vi "DeviceNet.vi"(0 "CloseVi?":bool) -> ()   [LabVIEW 2011]
uses:
  GlobalVariables.vi
panel:
  in  "DNET3_3":u8
  in  "DNET3_2":u8
  in  "DNET3_1":u8
  in  "DNET3_0":u8
  in  "DNET2_3":u8
  in  "DNET2_2":u8
  in  "DNET2_1":u8
  in  "DNET2_0":u8
  in  "DNET1_3":u8
  in  "DNET1_2":u8
  in  "DNET1_1":u8
  in  "DNET1_0":u8
  out "DNET3":string
  out "DNET2":string
  out "DNET1":string
  in  "close":bool
  in  "Reset":bool
  in  "HaltScanner":bool
  in  "DisableNetwork":bool
  in  "Fault":bool
  out "DnetPowerDetect":bool
  out "DupNodeFail":bool
  out "CommFailure":bool
  out "Autoverify":bool
  out "DeviceFailure":bool
  out "DisableNetwork":bool
  out "Fault":bool
  out "Run":bool
  in  "Run":bool
  in  "Reset":bool
  in  "HaltScanner":bool
  in  "DisableNetwork":bool
  in  "Fault":bool
  out "DnetPowerDetect":bool
  out "DupNodeFail":bool
  out "CommFailure":bool
  out "Autoverify":bool
  out "DeviceFailure":bool
  out "DisableNetwork":bool
  out "Fault":bool
  out "Run":bool
  in  "Run":bool
  in  "Reset":bool
  in  "HaltScanner":bool
  in  "DisableNetwork":bool
  in  "Fault":bool
  out "DnetPowerDetect":bool
  out "DupNodeFail":bool
  out "CommFailure":bool
  out "Autoverify":bool
  out "DeviceFailure":bool
  out "DisableNetwork":bool
  out "Fault":bool
  out "Run":bool
  in  "Run":bool
  # "DeviceNet 1"
  # "DeviceNet 2"
  # "DeviceNet 3"
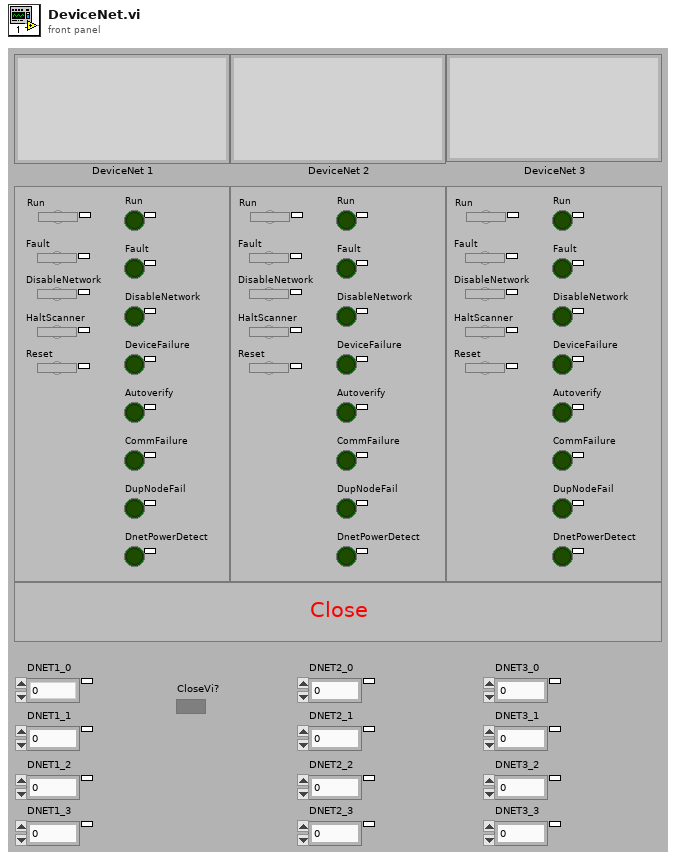
[diagram p1: front panel]
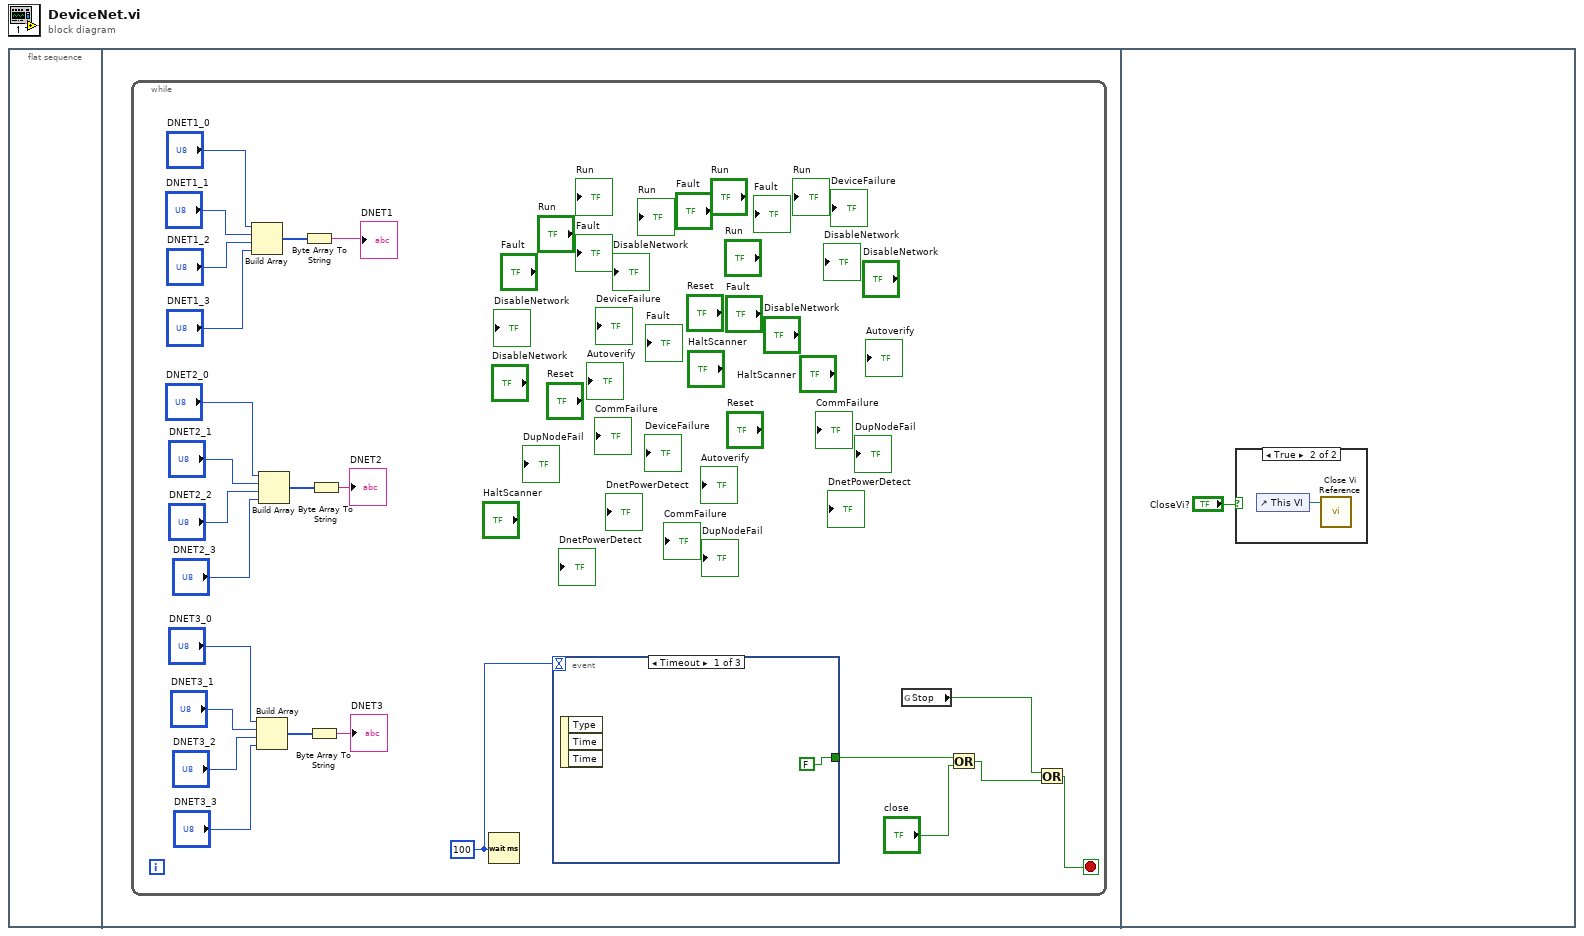
[diagram p0: block diagram]
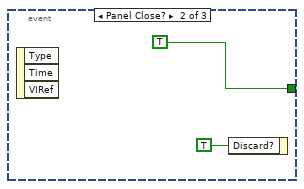
[diagram p2: hidden frame]
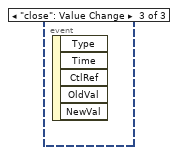
[diagram p3: hidden frame]
diagram:
  n1 = flat-sequence {
    frame #0 {
    }
    frame #1 {
      n2 = while {
        stop <- w6 stop-if-true
        w4 = 100
        n3 = Build Array("DNET1_0", "DNET1_1", "DNET1_2", "DNET1_3") -> (w20:u8[])
        n4 = Build Array("DNET3_0", "DNET3_1", "DNET3_2", "DNET3_3") -> (w17:u8[])
        n5 = Build Array("DNET2_0", "DNET2_1", "DNET2_2", "DNET2_3") -> (w18:u8[])
        n6 = Byte Array To String(unsigned byte array=w20) -> (string=→"DNET1":string)
        n7 = Byte Array To String(unsigned byte array=w17) -> (string=→"DNET3":string)
        n8 = Byte Array To String(unsigned byte array=w18) -> (string=→"DNET2":string)
        n9 = Wait (ms)(milliseconds to wait=w4) -> ()  [unwired: 1 out]
        n10 = event shown="[0] Timeout" {
          selector: _ -> [_ _ _]
          dyn-events: _ -> [_ _ _]
          timeout: w4 -> [_ _ _]
          tunnel: [FALSE ("y") TRUE ("y") _] -> w1
          event Timeout {
            n11 = event-data() -> ()  [unwired: 1 in, 3 out]
          }
          event Panel Close? {
            n12 = event-data() -> ()  [unwired: 1 in, 3 out]
            n13 = event-data("Discard?"=TRUE) -> ()  [unwired: 1 in, 1 out]
          }
          event "close": Value Change {
            n14 = event-data() -> ()  [unwired: 1 in, 5 out]
          }
        }
        n15 = global read "GlobalVariables.vi" "Stop"() -> (w5:bool)
        n16 = Or(x=w1, y="close") -> (x .or. y?=w3:bool)
        n17 = Or(x=w5, y=w3) -> (x .or. y?=w6:bool)
      }
    }
    frame #2 {
      n18 = case shown="True" "CloseVi?" {
        frame False {
        }
        frame True {
          n19 = control-ref of="This VI"() -> (w29:refnum<vi>)
          n20 = call "Close Vi Reference.vi"("reference"=w29) -> ()  [unwired: 9 in, 2 out]
        }
      }
    }
  }
